vi "OpenCreateReplace Dataset by Element Type.vi"(0 "HDF5 Location Ref":T2, 1 "Compression Level (0-disabled)":i32, 2 "Chunk size":i32[](array[numeric]), 5 "Dataset Path":string, 7 "Dataspace Dims":i32[](array[numeric]), 9 "Unlimited  dataset (F)":bool, 11 "error in (no error)":errorcluster, 12 "operation (open or create)":T1, 14 "Element Datatype":variant) -> (4 "HDF5 Location Ref":T2, 6 "HDF5 Dataset Ref":T2, 15 "error out":errorcluster)   [LabVIEW 2017]
uses:
  <vilib>/UPVI/lvhdf5/library.llb/HDF5 Ref.ctl
  <vilib>/UPVI/lvhdf5/dataset.llb/LVH5D Operation.ctl
panel:
  # "LVHDF5 Toolkit\nCopyright (c) 2005 - 2014 by Jason D. Sommerville\n\nThis use and distribution of this file is governed by the terms found in\n <user.lib>\\_lvhdf5\\LICENSE.txt"
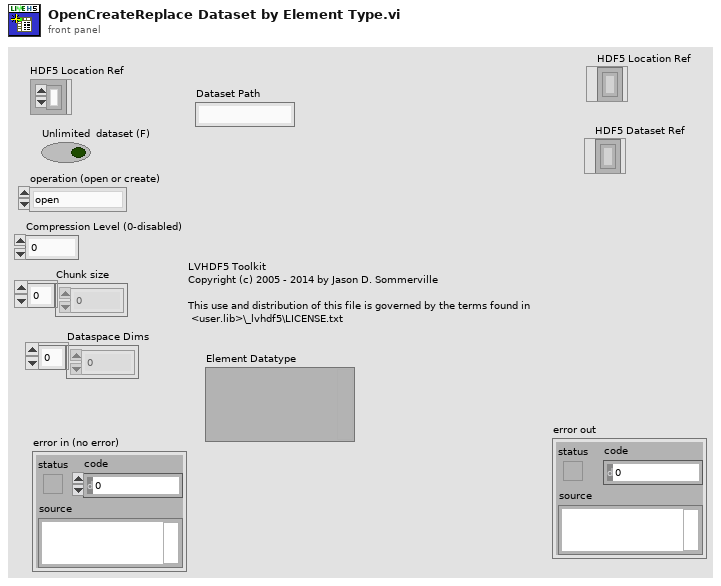
[diagram p1: front panel]
types:
  T1 = typedef "LVH5D Operation.ctl" = enum16{"open", "replace", "create", "open or create", "create or replace", "create or replace with confirmation"}
  T2 = typedef "HDF5 Ref.ctl" = refnum<k1>
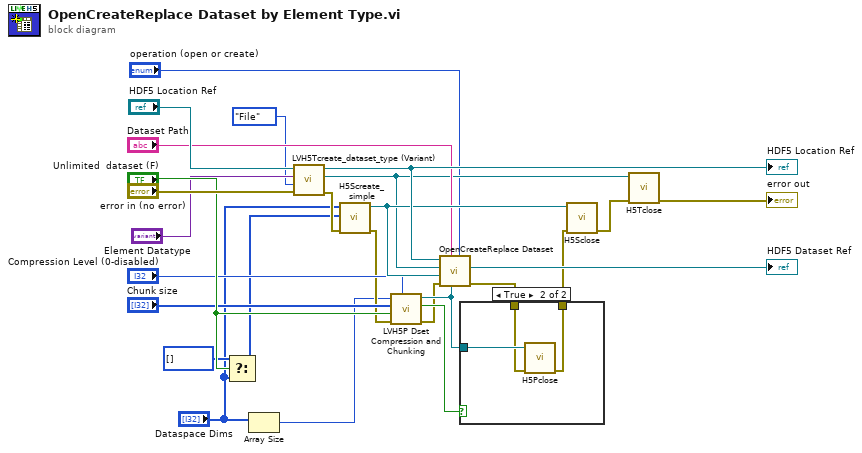
[diagram p0: block diagram]
diagram:
  n1 = Select(t=i32[] [], s="Unlimited  dataset (F)", f="Dataspace Dims") -> (s? t:f=w5:i32[])
  n2 = Array Size(array="Dataspace Dims") -> (size(s)=w1:i32)
  n3 = call <vilib>:"LVH5Tcreate_dataset_type (Variant).vi"("error in (no error)"="error in (no error)", "Type"=enum16{"File", "Memory"}."File", "Data"="Element Datatype", "HDF5 Ref"="HDF5 Location Ref") -> ("error out"=w14:errorcluster, "HDF5 Type Ref"=w6:T2, "HDF5 Ref out"=w25:T2)  [unwired: 3 in, 2 out]
  "HDF5 Location Ref" <- w25
  n4 = call <vilib>:"H5Screate_simple.vi"("error in (no error)"=w14, "Maximum Dimensions (unlimited)"=w5, "Dimensions"="Dataspace Dims") -> ("error out"=w15:errorcluster, "HDF5 Ref out"=w21:T2)  [unwired: 5 in]
  n5 = call <vilib>:"LVH5P Dset Compression and Chunking.vi"("Compression Level (0-disabled)"="Compression Level (0-disabled)", "error in (no error)"=w15, "Unlimited  dataset (F)"="Unlimited  dataset (F)", "Chunk size"="Chunk size", "Dataspace Rank"=w1) -> ("error out"=w10:errorcluster, "Created dcpl?"=w12:bool, "Dataset Creation Property List"=w11:T2)  [unwired: 4 in]
  n6 = call <vilib>:"OpenCreateReplace Dataset.vi"("operation (open or create)"="operation (open or create)", "HDF5 Property List Ref"=w11, "Dataset Path"="Dataset Path", "error in (no error)"=w10, "HDF5 Dataspace Ref"=w21, "HDF5 Datatype Ref"=w6, "HDF5 Ref"=w25) -> ("error out"=w9:errorcluster, "HDF5 Dataset Ref"=→"HDF5 Dataset Ref":T2)  [unwired: 2 in, 1 out]
  n7 = case shown="True" w12 {
    tunnel: w11 -> [_ w30]
    tunnel: w9 -> [w27 w29]
    tunnel: [w27 w28] -> w8
    frame False {
    }
    frame True {
      n8 = call <vilib>:"H5Pclose.vi"("error in (no error)"=w29, "HDF5 Property Ref"=w30) -> ("error out"=w28:errorcluster)  [unwired: 7 in]
    }
  }
  n9 = call <vilib>:"H5Sclose.vi"("error in (no error)"=w8, "HDF5 Dataspace Ref"=w21) -> ("error out"=w7:errorcluster)  [unwired: 7 in]
  n10 = call <vilib>:"H5Tclose.vi"("error in (no error)"=w7, "HDF5 Datatype Ref"=w6) -> ("error out"=→"error out":errorcluster)  [unwired: 7 in]
